vi "AMZ_S3_AWS Credentials FG.vi"(6 "Set?":bool, 8 "error in (no error)":errorcluster, 11 "AWS Credentials in":T1) -> (0 "error out":errorcluster, 3 "AWS Credentials":T1)   [LabVIEW 2015, in "LV Interface for Amazon S3.lvlib"]
uses:
  LV Interface for Amazon S3.lvlib
  Typedefs/AMZ_S3_AWS Credentials.ctl
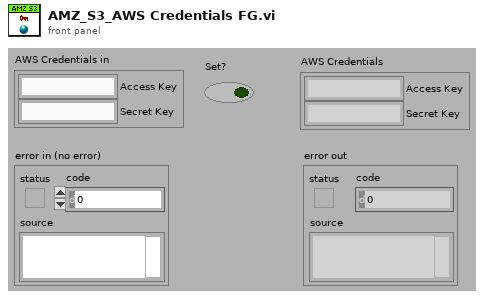
[diagram p1: front panel]
types:
  T1 = typedef "LV Interface for Amazon S3.lvlib/AMZ_S3_AWS Credentials.ctl" = cluster{"Access Key":string, "Secret Key":string}
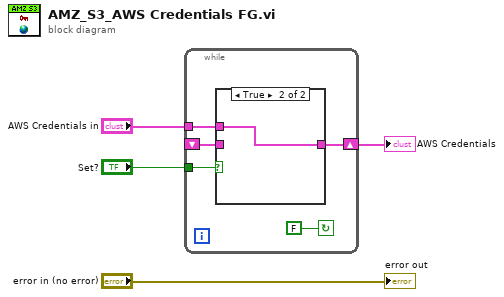
[diagram p0: block diagram]
diagram:
  n1 = while {
    tunnel: "AWS Credentials in" -> [w7]
    tunnel: "Set?" -> [w8]
    shift-right: [w6] -> w2
    shift-left: _ -> [w5]
    stop <- FALSE continue-if-true
    n2 = case shown="True" w8 {
      tunnel: w7 -> [_ w11]
      tunnel: [w10 w11] -> w6
      tunnel: w5 -> [w10 _]
      frame False {
      }
      frame True {
      }
    }
  }
  "AWS Credentials" <- w2
  "error out" <- "error in (no error)"
